vi "UICtrls_Write_Index_Array.vi"(8 "error in":errorcluster, 9 "Control Value":variant[](array[variant]), 10 "Index":i32[](array[numeric]), 11 "UI Ref cluster in":T1) -> (0 "error out":errorcluster, 3 "UI Ref cluster out":T1)   [LabVIEW 2025]
doc: "Write new value to all Controls by index if found"
uses:
  UI_Manager/UI_Manager.lvclass
  Controls/UI_Ref_Cluster.ctl
  UI_Manager.lvlib
  <vilib>/Utility/Data Type/Type Definitions/Data Type.ctl
  <vilib>/Utility/Data Type/NI_Data Type.lvlib
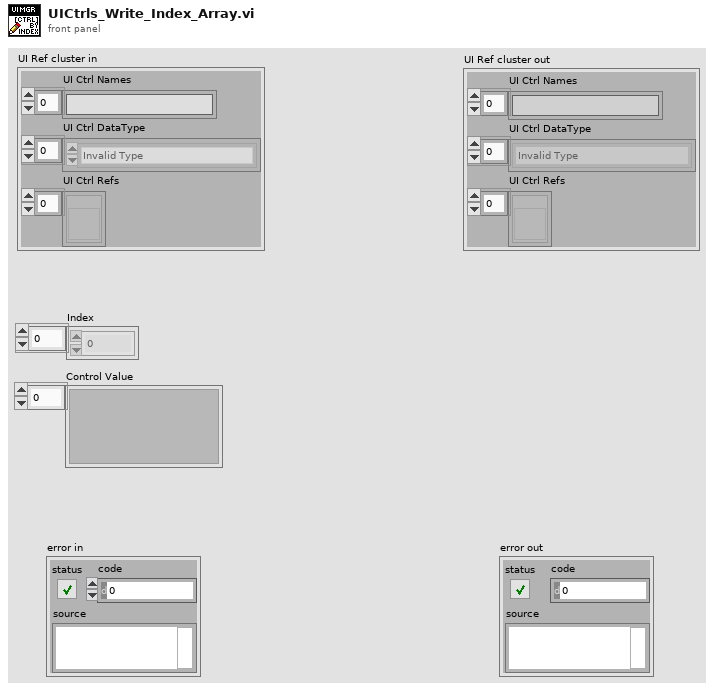
[diagram p1: front panel]
types:
  T1 = typedef "UI_Manager.lvlib/UI_Ref_Cluster.ctl" = cluster{"UI Ctrl Names":string[], "UI Ctrl DataType":T2[], "UI Ctrl Refs":refnum<vi>[]}
  T2 = typedef "NI_Data Type.lvlib/Data Type.ctl" = enum8{"Invalid Type", "Void", "I8", "I16", "I32", "I64", "U8", "U16", "U32", "U64", "Single Float", "Double Float", "Extended Float", "Single Complex", "Double Complex", "Extended Complex", "Enum U8", "Enum U16", "Enum U32", "Enum U64", "Single Float With Unit", "Double Float With Unit", "Extended Float With Unit", "Single Complex with Unit", "Double Complex with Unit", "Extended Complex with Unit", "Boolean", "String", "Path", "Picture", "Tag", "Array", "Cluster", "Variant", "LV Variant", "Waveform", "Timestamp", "Digital Waveform", "Digital Data", "ExpressData", "Refnum", "External Data", "VI", "Poly VI", "LabVIEW Class Instance", "Fixed Point", "Set Collection", "Map Collection"}
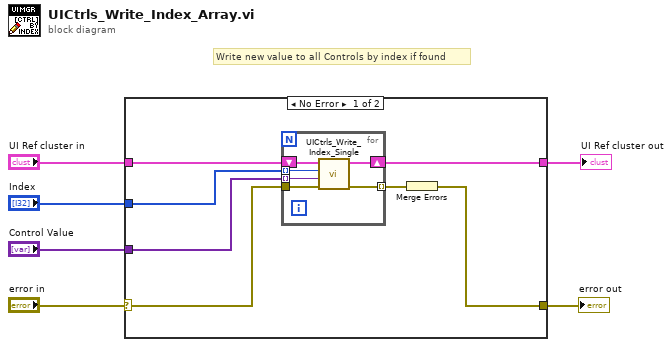
[diagram p0: block diagram]
diagram:
  # "Write new value to all Controls by index if found"
  n1 = case shown="No Error" "error in" {
    selector: "error in" -> [w11 w21]
    tunnel: [w7 w21] -> w6
    tunnel: "Control Value" -> [w8 _]
    tunnel: [w12 w20] -> w3
    tunnel: "UI Ref cluster in" -> [w13 w20]
    tunnel: "Index" -> [w9 _]
    frame No Error {
      n2 = for {
        tunnel: w9 -> [w15] mode=indexing
        tunnel: w8 -> [w14] mode=indexing
        shift-right: [w18] -> w12
        shift-left: w13 -> [w19]
        tunnel: w11 -> [w17]
        tunnel: [w16] -> w10 mode=indexing
        n3 = call "UICtrls_Write_Index_Single.vi"("error in"=w17, "Control Value"=w14, "Index"=w15, "UI Ref cluster in"=w19) -> ("error out"=w16:errorcluster, "UI Ref cluster out"=w18:T1)  [unwired: 6 in]
      }
      n4 = Merge Errors(w10) -> (w7:errorcluster)
    }
    frame Error {
    }
  }
  "error out" <- w6
  "UI Ref cluster out" <- w3
